vi "Tree Get Default.vi"(8 "error in (no error)":errorcluster, 11 "Tree DVR in":refnum<data-value>) -> (0 "error out":errorcluster, 2 "Node out":refnum<data-value>, 3 "Tree DVR out":refnum<data-value>)   [LabVIEW 2012, in "MDSplus.lvlib"]
doc: "Get the TreeNode for the default node."
uses:
  <vilib>/MDSplus/Library/MDSplus.lvlib
  <vilib>/MDSplus/Classes/Tree_Class/Tree.lvclass
  <vilib>/MDSplus/Classes/Data_Class/TreeNode_Class/TreeNode.lvclass
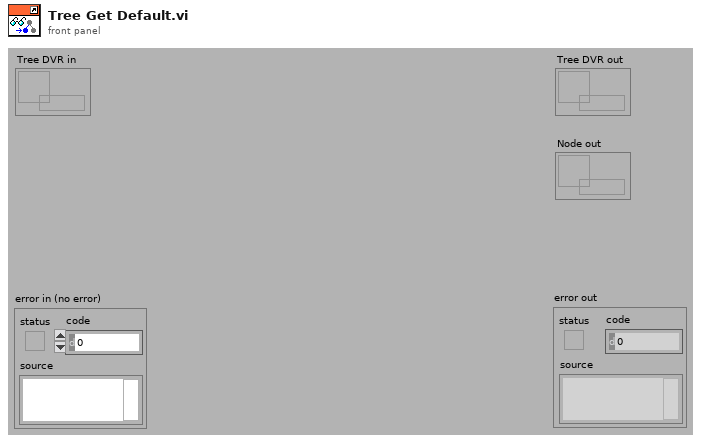
[diagram p1: front panel]
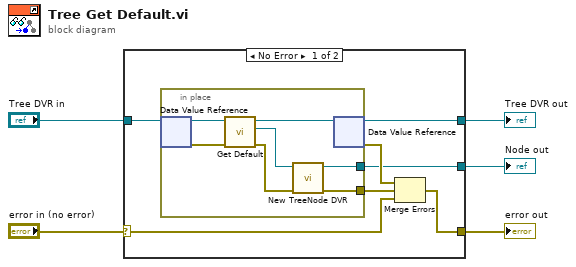
[diagram p0: block diagram]
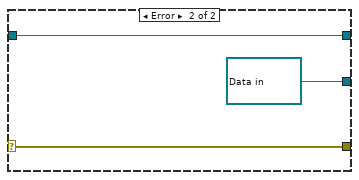
[diagram p2: hidden frame]
diagram:
  n1 = case shown="No Error" "error in (no error)" {
    selector: "error in (no error)" -> [w11 w22]
    tunnel: "Tree DVR in" -> [w12 w21]
    tunnel: [w9 w22] -> w5
    tunnel: [w8 w21] -> w2
    tunnel: [w7 refnum<data-value> refnum ("TreeNode DVR out")] -> w1
    frame No Error {
      n2 = in-place {
        in-place-border: [w13] -> w6
        in-place-border: [w15] -> w7
        n3 = in-place-dvr #1(w12) -> (w19:refnum<class "Tree.lvclass">, w17:errorcluster)
        n4 = call-dynamic "Get Default.vi"("error in (no error)"=w17, "Tree in"=w19) -> ("error out"=w14:errorcluster, "Node out"=w16:refnum<class "TreeNode.lvclass">, "Tree out"=w18:refnum<class "Tree.lvclass">)  [unwired: 7 in]
        n5 = call <vilib>:"New TreeNode DVR.vi"("error in (no error)"=w14, "TreeNode in"=w16) -> ("error out"=w13:errorcluster, "TreeNode DVR out"=w15:refnum<data-value>)  [unwired: 8 in]
        n6 = in-place-dvr #1(w18) -> (w8:refnum<data-value>, w10:errorcluster)
      }
      n7 = Merge Errors(w10, w6, w11) -> (w9:errorcluster)
    }
    frame Error {
    }
  }
  "error out" <- w5
  "Tree DVR out" <- w2
  "Node out" <- w1
